vi "Close.vi"(8 "error in":errorcluster, 11 "HSU MCU V2 Monitor CFG in":refnum<class "HSU MCU V2 CFG.lvclass">) -> (0 "error out":errorcluster, 3 "HSU MCU V2 Monitor CFG out":refnum<class "HSU MCU V2 CFG.lvclass">)   [LabVIEW 2023, in "HSU MCU V2 CFG.lvclass"]
uses:
  HSU MCU V2 CFG.lvclass
  Configurations/CFG Base/CFG Base.lvclass
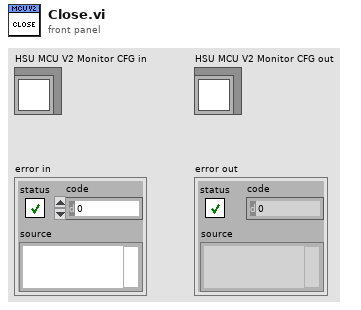
[diagram p1: front panel]
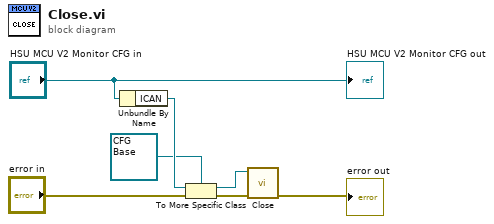
[diagram p0: block diagram]
diagram:
  n1 = Unbundle By Name("HSU MCU V2 Monitor CFG in") -> ("ICAN"=w5:refnum<class "ICAN.lvclass">)
  n2 = To More Specific Class(target class=refnum<class "CFG Base.lvclass"> refnum ("HAL.lvlib:CFG Base.lvclass"), reference=w5, error in="error in") -> (specific class reference=w2:refnum<class "CFG Base.lvclass">, error out=w4:errorcluster)
  n3 = call-dynamic "Close.vi"("error in"=w4, "CFG Base in"=w2) -> ("error out"=→"error out":errorcluster)  [unwired: 8 in, 1 out]
  "HSU MCU V2 Monitor CFG out" <- "HSU MCU V2 Monitor CFG in"
